vi "Remove Device from Stack.vi"(8 "error in (no error)":errorcluster, 10 "Device in":refnum<class "Device.lvclass">, 11 "IP Connection in":refnum<class "IP Connection.lvclass">) -> (0 "error out":errorcluster, 3 "IP Connection out":refnum<class "IP Connection.lvclass">)   [LabVIEW 2011, in "Tinkerforge.lvlib" / "IP Connection.lvclass"]
doc: "This VI removes <B>Device</B> from the stack."
uses:
  IP Connection.lvclass
  Device/Device.lvclass
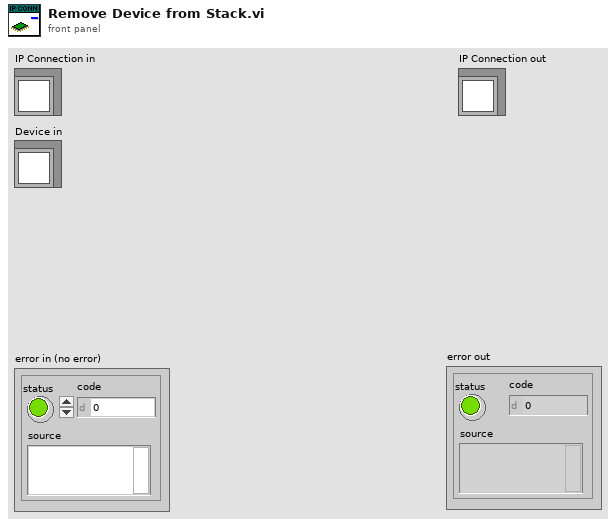
[diagram p1: front panel]
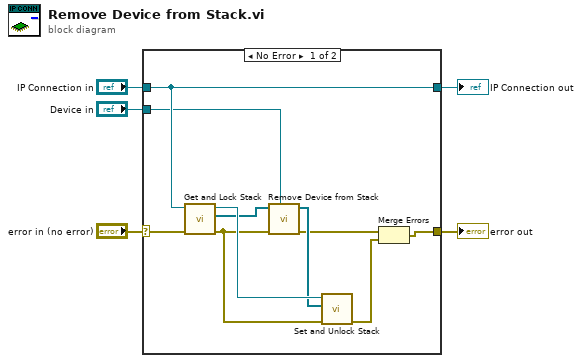
[diagram p0: block diagram]
diagram:
  n1 = case shown="No Error" "error in (no error)" {
    selector: "error in (no error)" -> [w14 w17]
    tunnel: [w15 w17] -> w4
    tunnel: [w13 w16] -> w2
    tunnel: "IP Connection in" -> [w13 w16]
    tunnel: "Device in" -> [w6 _]
    frame No Error {
      n2 = call "Get and Lock Stack.vi"("error in (no error)"=w14, "IP Connection in"=w13) -> ("error out"=w10:errorcluster, "Stack"=w7:refnum<class "Device.lvclass">[], "IP Connection out"=w11:refnum<class "IP Connection.lvclass">)  [unwired: 7 in]
      n3 = call "Remove Device from Stack.vi"("Device"=w6, "error in (no error)"=w10, "Stack in"=w7) -> ("error out"=w8:errorcluster, "Stack out"=w9:refnum<class "Device.lvclass">[])  [unwired: 7 in]
      n4 = call "Set and Unlock Stack.vi"("error in (no error)"=w10, "Stack"=w9, "IP Connection in"=w11) -> ("error out"=w12:errorcluster)  [unwired: 7 in, 1 out]
      n5 = Merge Errors(w8, w12) -> (w15:errorcluster)
    }
    frame Error {
    }
  }
  "error out" <- w4
  "IP Connection out" <- w2
